vi "test.vi"() -> ()   [LabVIEW 2010]
panel:
  out "Plot":dynamicdata(graph)
  out "Numeric":i32
  out "Resistance (MOhm)":dbl
  in  "data 2":dbl
  in  "stop":bool
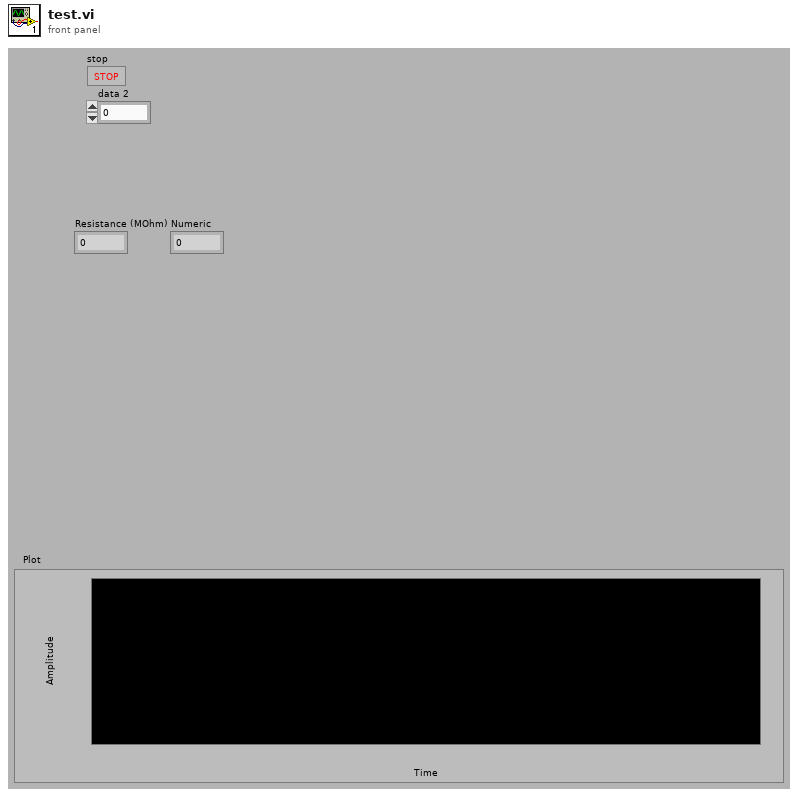
[diagram p1: front panel]
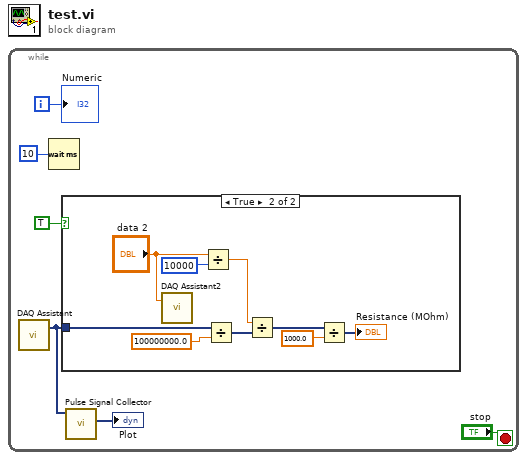
[diagram p0: block diagram]
diagram:
  n1 = while {
    i -> [w4]
    stop <- "stop" stop-if-true
    n2 = call "DAQ Assistant"() -> ("data"=w2:dynamicdata)  [unwired: 17 in, 2 out]
    n3 = Wait (ms)(milliseconds to wait=u32 10) -> ()  [unwired: 1 out]
    n4 = case shown="True" TRUE {
      tunnel: w2 -> [_ w13]
      frame False {
      }
      frame True {
        n5 = call "DAQ Assistant2"("data"="data 2") -> ()  [unwired: 17 in, 2 out]
        n6 = Divide(x="data 2", y=10000) -> (x/y=w11:dbl)
        n7 = Divide(x=w13, y=100000000.0) -> (x/y=w10:dynamicdata)
        n8 = Divide(x=w11, y=w10) -> (x/y=w9:dynamicdata)
        n9 = Divide(x=w9, y=1000.0) -> (x/y=→"Resistance (MOhm)":dynamicdata)
      }
    }
    n10 = call "Pulse Signal Collector"("Signals"=w2) -> ("Collected Signals"=→"Plot":dynamicdata)  [unwired: 9 in, 1 out]
    "Numeric" <- w4
  }
